vi "Retrieve Message with Options.vi"(4 "error in":errorcluster, 5 "delete from server (Y)?":bool=TRUE, 6 "message #":i32 min=0, 7 "connection ID in":refnum<k5>) -> (0 "error out":errorcluster, 2 "Message":string="\r\n", 3 "connection ID out":refnum<k5>)   [LabVIEW 2012]
doc: "This mid-level VI retrieves the specified message from a mail server, deleting the message by default unless the user specifies otherwise."
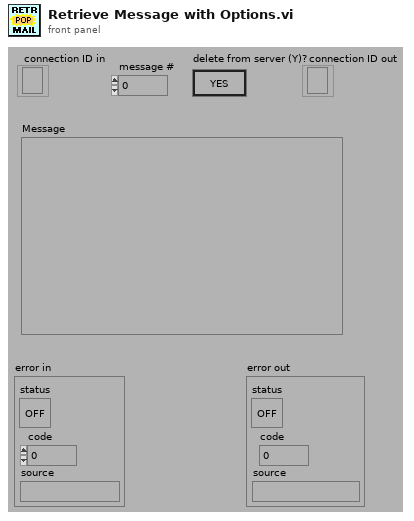
[diagram p1: front panel]
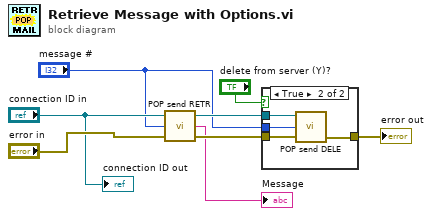
[diagram p0: block diagram]
diagram:
  n1 = call "POP send RETR.vi"("error in"="error in", "MSG number"="message #", "connection ID in"="connection ID in") -> ("error out"=w4:errorcluster, "RETR response"=→"Message":string, "connection ID out"=w3:refnum<k5>)
  n2 = case shown="True" "delete from server (Y)?" {
    tunnel: w4 -> [w9 w13]
    tunnel: [w9 w12] -> w7
    tunnel: w3 -> [_ w11]
    tunnel: "message #" -> [_ w10]
    frame False {
    }
    frame True {
      n3 = call "POP send DELE.vi"("error in"=w13, "MSG number"=w10, "connection ID in"=w11) -> ("error out"=w12:errorcluster)  [unwired: 2 out]
    }
  }
  "error out" <- w7
  "connection ID out" <- "connection ID in"
